vi "readAnalogTriggered.vi"(4 "Maximum Value":dbl=10.0 format="%0.2f", 6 "Minimum Value":dbl=-10.0 format="%0.2f", 8 "Physical Channel":refnum<k21>="Dev0/Ai1:0", 9 "Sample Rate":dbl=600.0 caption="Sample Rate (Hz)", 10 "clock source":i32(ring) items=["OnboardClock", "ExternalClock", "NoClock"], 11 "stop":bool) -> (3 "data":dbl[](array[numeric]))   [LabVIEW 2011]
uses:
  <vilib>/Utility/error.llb/DialogType.ctl
  <vilib>/ULx/Create Channel.llb/ULx Create Channel (AI-Voltage-Basic).vi
  <vilib>/ULx/Timing.llb/ULx Timing (Sample Clock).vi
  <vilib>/ULx/Trigger.llb/ULx Basic Trigger (Analog Edge).vi
  <vilib>/ULx/Read.llb/ULx Read (Analog 1D DBL NChan 1Samp).vi
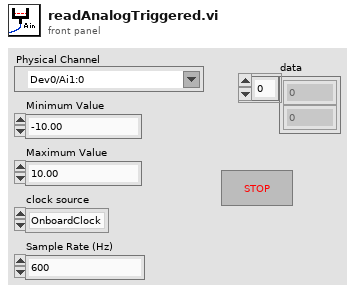
[diagram p1: front panel]
types:
  T1 = typedef "DialogType.ctl" = u16
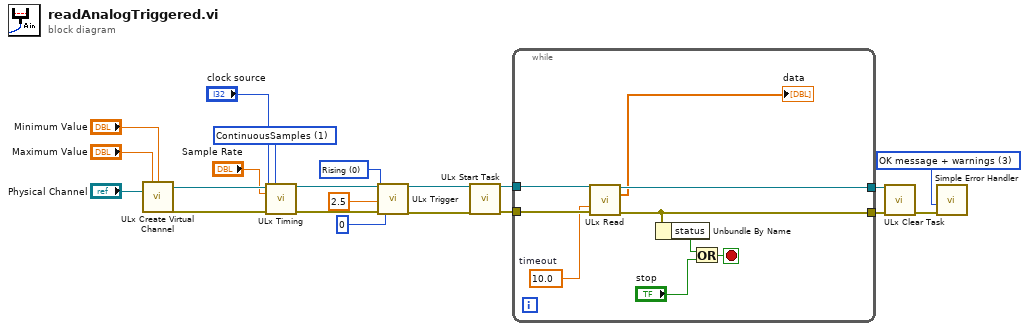
[diagram p0: block diagram]
diagram:
  w3 = 0 items=["Rising", "Falling"] ("slope")
  w13 = 1 items=["FiniteSamples", "ContinuousSamples"] ("sample mode")
  w14 = T1 3 items=["no dialog", "OK message", "continue or stop message", "OK message + warnings", "continue/stop + warnings"] ("type of dialog (OK msg:1)")
  n1 = call-poly <vilib>:"ULx Create Virtual Channel.vi"("maximum value"="Maximum Value", "minimum value"="Minimum Value", "physical channels"="Physical Channel") -> ("task out"=w18:refnum<k24>, "error out"=w21:errorcluster)  [unwired: 11 in]
  n2 = call-poly <vilib>:"ULx Timing.vi"("task in"=w18, "sample mode"=w13, "rate"="Sample Rate", "clock source"="clock source", "error in"=w21) -> ("task out"=w7:refnum<k24>, "error out"=w5:errorcluster)  [unwired: 9 in]
  n3 = call-poly <vilib>:"ULx Trigger.vi"("task in"=w7, "slope"=w3, "level"=2.5, "error in"=w5, "pretrigger samples per channel"=u32 0) -> ("task out"=w6:refnum<k24>, "error out"=w4:errorcluster)  [unwired: 13 in]
  n4 = call <vilib>:"ULx Start Task.vi"("task in"=w6, "error in"=w4) -> ("task out"=w17:refnum<k24>, "error out"=w20:errorcluster)  [unwired: 12 in]
  n5 = while {
    tunnel: w20 -> [w30]
    tunnel: w17 -> [w29]
    tunnel: [w28] -> w16
    tunnel: [w27] -> w15
    stop <- w25 stop-if-true
    w23 = 10.0  # timeout
    n6 = call-poly <vilib>:"ULx Read.vi"("task in"=w29, "timeout"=w23, "error in"=w30) -> ("task out"=w28:refnum<k24>, "data"=→"data":dbl[], "error out"=w27:errorcluster)  [unwired: 10 in]
    n7 = Unbundle By Name(w27) -> ("status"=w26:bool)
    n8 = Or(x=w26, y="stop") -> (x .or. y?=w25:bool)
  }
  n9 = call <vilib>:"ULx Clear Task.vi"("task in"=w16, "error in"=w15) -> ("error out"=w19:errorcluster)  [unwired: 13 in]
  n10 = call <vilib>:"Simple Error Handler.vi"("type of dialog (OK msg:1)"=w14, "error in (no error)"=w19) -> ()  [unwired: 3 in, 5 out]
